vi "CAEN_HVChannel.Create DIM Services.vi"(0 "i ref in":refnum<vi>, 5 "error in":errorcluster) -> (14 "i ref out":refnum<vi>, 19 "error out":errorcluster)   [LabVIEW 2014, in "CAEN_HVChannel.lvlib"]
doc: "This method is used to define the events the object will listen to. Add your own events here."
uses:
  CAEN_HVChannel.lvlib
  CSlibraries-extern/DimLVEvent/LVDimInterface/LVDimInterface.lvlib
  CS_Core/CSSystem/CSSystemLib/CSSystemLib.lvlib
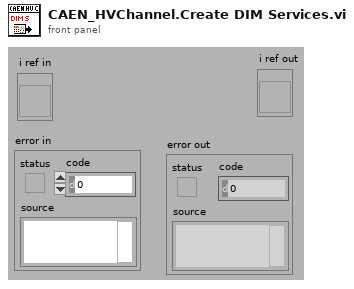
[diagram p1: front panel]
types:
  T1 = typedef "CAEN_HVChannel.lvlib/CAEN_HVChannel.i attribute.ctl" = cluster{"Channel Array":cluster{"Logical Name":string, "Address":string, "error in (no error)":errorcluster, "Name":cluster{"Name":string, "DIM Status":cluster{"no link":bool, "quality":i32, "Time Stamp":timestamp}}, "Status":cluster{"Status":i16, "DIM Status":cluster{"no link":bool, "quality":i32, "Time Stamp":timestamp}}, "V0Set":cluster{"V0Set#EU":cluster{"V0Set#EU":string, "DIM Status":cluster{"no link":bool, "quality":i32, "Time Stamp":timestamp}}, "V0Set":cluster{"V0Set":dbl, "DIM Status":cluster{"no link":bool, "quality":i32, "Time Stamp":timestamp}}, "V0Set#HighEU":cluster{"V0Set#HighEU":dbl, "DIM Status":cluster{"no link":bool, "quality":i32, "Time Stamp":timestamp}}, "V0Set#LowEU":cluster{"V0Set#LowEU":dbl, "DIM Status":cluster{"no link":bool, "quality":i32, "Time Stamp":timestamp}}, "V0Set#Multiplier":dbl}, "I0Set":cluster{"I0Set#EU":cluster{"I0Set#EU":string, "DIM Status":cluster{"no link":bool, "quality":i32, "Time Stamp":timestamp}}, "I0Set":cluster{"I0Set":dbl, "DIM Status":cluster{"no link":bool, "quality":i32, "Time Stamp":timestamp}}, "I0Set#HighEU":cluster{"I0Set#HighEU":dbl, "DIM Status":cluster{"no link":bool, "quality":i32, "Time Stamp":timestamp}}, "I0Set#LowEU":cluster{"I0Set#LowEU":dbl, "DIM Status":cluster{"no link":bool, "quality":i32, "Time Stamp":timestamp}}, "I0Set#Multiplier":dbl}, "V1Set":cluster{"V1Set#EU":cluster{"V1Set#EU":string, "DIM Status":cluster{"no link":bool, "quality":i32, "Time Stamp":timestamp}}, "V1Set":cluster{"V1Set":dbl, "DIM Status":cluster{"no link":bool, "quality":i32, "Time Stamp":timestamp}}, "V1Set#HighEU":cluster{"V1Set#HighEU":dbl, "DIM Status":cluster{"no link":bool, "quality":i32, "Time Stamp":timestamp}}, "V1Set#LowEU":cluster{"V1Set#LowEU":dbl, "DIM Status":cluster{"no link":bool, "quality":i32, "Time Stamp":timestamp}}, "V1Set#Multiplier":dbl}, "I1Set":cluster{"I1Set#EU":cluster{"I1Set#EU":string, "DIM Status":cluster{"no link":bool, "quality":i32, "Time Stamp":timestamp}}, "I1Set":cluster{"I1Set":dbl, "DIM Status":cluster{"no link":bool, "quality":i32, "Time Stamp":timestamp}}, "I1Set#HighEU":cluster{"I1Set#HighEU":dbl, "DIM Status":cluster{"no link":bool, "quality":i32, "Time Stamp":timestamp}}, "I1Set#LowEU":cluster{"I1Set#LowEU":dbl, "DIM Status":cluster{"no link":bool, "quality":i32, "Time Stamp":timestamp}}, "I1Set#Multiplier":dbl}, "RUp":cluster{"RUp#EU":cluster{"RUp#EU":string, "DIM Status":cluster{"no link":bool, "quality":i32, "Time Stamp":timestamp}}, "RUp":cluster{"RUp":dbl, "DIM Status":cluster{"no link":bool, "quality":i32, "Time Stamp":timestamp}}, "RUp#HighEU":cluster{"RUp#HighEU":dbl, "DIM Status":cluster{"no link":bool, "quality":i32, "Time Stamp":timestamp}}, "RUp#LowEU":cluster{"RUp#LowEU":dbl, "DIM Status":cluster{"no link":bool, "quality":i32, "Time Stamp":timestamp}}, "RUp#Multiplier":dbl}, "RDWn":cluster{"RDWn#EU":cluster{"RDWn#EU":string, "DIM Status":cluster{"no link":bool, "quality":i32, "Time Stamp":timestamp}}, "RDWn":cluster{"RDWn":dbl, "DIM Status":cluster{"no link":bool, "quality":i32, "Time Stamp":timestamp}}, "RDWn#HighEU":cluster{"RDWn#HighEU":dbl, "DIM Status":cluster{"no link":bool, "quality":i32, "Time Stamp":timestamp}}, "RDWn#LowEU":cluster{"RDWn#LowEU":dbl, "DIM Status":cluster{"no link":bool, "quality":i32, "Time Stamp":timestamp}}, "RDWn#Multiplier":dbl}, "Trip":cluster{"Trip#EU":cluster{"Trip#EU":string, "DIM Status":cluster{"no link":bool, "quality":i32, "Time Stamp":timestamp}}, "Trip":cluster{"Trip":dbl, "DIM Status":cluster{"no link":bool, "quality":i32, "Time Stamp":timestamp}}, "Trip#HighEU":cluster{"Trip#HighEU":dbl, "DIM Status":cluster{"no link":bool, "quality":i32, "Time Stamp":timestamp}}, "Trip#LowEU":cluster{"Trip#LowEU":dbl, "DIM Status":cluster{"no link":bool, "quality":i32, "Time Stamp":timestamp}}, "Trip#Multiplier":dbl}, "SVMax":cluster{"SVMax#EU":cluster{"SVMax#EU":string, "DIM Status":cluster{"no link":bool, "quality":i32, "Time Stamp":timestamp}}, "SVMax":cluster{"SVMax":dbl, "DIM Status":cluster{"no link":bool, "quality":i32, "Time Stamp":timestamp}}, "SVMax#HighEU":cluster{"SVMax#HighEU":dbl, "DIM Status":cluster{"no link":bool, "quality":i32, "Time Stamp":timestamp}}, "SVMax#LowEU":cluster{"SVMax#LowEU":dbl, "DIM Status":cluster{"no link":bool, "quality":i32, "Time Stamp":timestamp}}, "SVMax#Multiplier":dbl}, "VMon":cluster{"VMon#EU":cluster{"VMon#EU":string, "DIM Status":cluster{"no link":bool, "quality":i32, "Time Stamp":timestamp}}, "VMon":cluster{"VMon":dbl, "DIM Status":cluster{"no link":bool, "quality":i32, "Time Stamp":timestamp}}, "VMon#HighEU":cluster{"VMon#HighEU":dbl, "DIM Status":cluster{"no link":bool, "quality":i32, "Time Stamp":timestamp}}, "VMon#LowEU":cluster{"VMon#LowEU":dbl, "DIM Status":cluster{"no link":bool, "quality":i32, "Time Stamp":timestamp}}, "VMon#Multiplier":dbl}, "IMon":cluster{"IMon#EU":cluster{"IMon#EU":string, "DIM Status":cluster{"no link":bool, "quality":i32, "Time Stamp":timestamp}}, "IMon":cluster{"IMon":dbl, "DIM Status":cluster{"no link":bool, "quality":i32, "Time Stamp":timestamp}}, "IMon#HighEU":cluster{"IMon#HighEU":dbl, "DIM Status":cluster{"no link":bool, "quality":i32, "Time Stamp":timestamp}}, "IMon#LowEU":cluster{"IMon#LowEU":dbl, "DIM Status":cluster{"no link":bool, "quality":i32, "Time Stamp":timestamp}}, "IMon#Multiplier":dbl}, "TripInt":cluster{"TripInt#EU":cluster{"TripInt#EU":string, "DIM Status":cluster{"no link":bool, "quality":i32, "Time Stamp":timestamp}}, "TripInt":cluster{"TripInt":dbl, "DIM Status":cluster{"no link":bool, "quality":i32, "Time Stamp":timestamp}}, "TripInt#HighEU":cluster{"TripInt#HighEU":dbl, "DIM Status":cluster{"no link":bool, "quality":i32, "Time Stamp":timestamp}}, "TripInt#LowEU":cluster{"TripInt#LowEU":dbl, "DIM Status":cluster{"no link":bool, "quality":i32, "Time Stamp":timestamp}}, "TripInt#Multiplier":dbl}, "TripExt":cluster{"TripExt#EU":cluster{"TripExt#EU":string, "DIM Status":cluster{"no link":bool, "quality":i32, "Time Stamp":timestamp}}, "TripExt":cluster{"TripExt":dbl, "DIM Status":cluster{"no link":bool, "quality":i32, "Time Stamp":timestamp}}, "TripExt#HighEU":cluster{"TripExt#HighEU":dbl, "DIM Status":cluster{"no link":bool, "quality":i32, "Time Stamp":timestamp}}, "TripExt#LowEU":cluster{"TripExt#LowEU":dbl, "DIM Status":cluster{"no link":bool, "quality":i32, "Time Stamp":timestamp}}, "TripExt#Multiplier":dbl}, "Pw":cluster{"Pw":cluster{"Pw":bool, "DIM Status":cluster{"no link":bool, "quality":i32, "Time Stamp":timestamp}}, "Pw#CoClose":cluster{"Pw#CoClose":string, "DIM Status":cluster{"no link":bool, "quality":i32, "Time Stamp":timestamp}}, "Pw#CoOpen":cluster{"Pw#CoOpen":string, "DIM Status":cluster{"no link":bool, "quality":i32, "Time Stamp":timestamp}}}, "POn":cluster{"POn":cluster{"POn":bool, "DIM Status":cluster{"no link":bool, "quality":i32, "Time Stamp":timestamp}}, "POn#CoClose":cluster{"POn#CoClose":string, "DIM Status":cluster{"no link":bool, "quality":i32, "Time Stamp":timestamp}}, "POn#CoOpen":cluster{"POn#CoOpen":string, "DIM Status":cluster{"no link":bool, "quality":i32, "Time Stamp":timestamp}}}, "PDwn":cluster{"PDwn":cluster{"PDwn":bool, "DIM Status":cluster{"no link":bool, "quality":i32, "Time Stamp":timestamp}}, "PDwn#CoClose":cluster{"PDwn#CoClose":string, "DIM Status":cluster{"no link":bool, "quality":i32, "Time Stamp":timestamp}}, "PDwn#CoOpen":cluster{"PDwn#CoOpen":string, "DIM Status":cluster{"no link":bool, "quality":i32, "Time Stamp":timestamp}}}, "DIM Service IDs":cluster{"nomV1Set":i32, "nomI1Set":i32, "nomTrip":i32, "nomSVMax":i32, "nomPOn":i32, "nomPDwn":i32, "nomTripInt":i32, "nomTripExt":i32}}[], "VoltageInRangeBand":dbl}
  T2 = cluster{"Logical Name":string, "Address":string, "error in (no error)":errorcluster, "Name":cluster{"Name":string, "DIM Status":cluster{"no link":bool, "quality":i32, "Time Stamp":timestamp}}, "Status":cluster{"Status":i16, "DIM Status":cluster{"no link":bool, "quality":i32, "Time Stamp":timestamp}}, "V0Set":cluster{"V0Set#EU":cluster{"V0Set#EU":string, "DIM Status":cluster{"no link":bool, "quality":i32, "Time Stamp":timestamp}}, "V0Set":cluster{"V0Set":dbl, "DIM Status":cluster{"no link":bool, "quality":i32, "Time Stamp":timestamp}}, "V0Set#HighEU":cluster{"V0Set#HighEU":dbl, "DIM Status":cluster{"no link":bool, "quality":i32, "Time Stamp":timestamp}}, "V0Set#LowEU":cluster{"V0Set#LowEU":dbl, "DIM Status":cluster{"no link":bool, "quality":i32, "Time Stamp":timestamp}}, "V0Set#Multiplier":dbl}, "I0Set":cluster{"I0Set#EU":cluster{"I0Set#EU":string, "DIM Status":cluster{"no link":bool, "quality":i32, "Time Stamp":timestamp}}, "I0Set":cluster{"I0Set":dbl, "DIM Status":cluster{"no link":bool, "quality":i32, "Time Stamp":timestamp}}, "I0Set#HighEU":cluster{"I0Set#HighEU":dbl, "DIM Status":cluster{"no link":bool, "quality":i32, "Time Stamp":timestamp}}, "I0Set#LowEU":cluster{"I0Set#LowEU":dbl, "DIM Status":cluster{"no link":bool, "quality":i32, "Time Stamp":timestamp}}, "I0Set#Multiplier":dbl}, "V1Set":cluster{"V1Set#EU":cluster{"V1Set#EU":string, "DIM Status":cluster{"no link":bool, "quality":i32, "Time Stamp":timestamp}}, "V1Set":cluster{"V1Set":dbl, "DIM Status":cluster{"no link":bool, "quality":i32, "Time Stamp":timestamp}}, "V1Set#HighEU":cluster{"V1Set#HighEU":dbl, "DIM Status":cluster{"no link":bool, "quality":i32, "Time Stamp":timestamp}}, "V1Set#LowEU":cluster{"V1Set#LowEU":dbl, "DIM Status":cluster{"no link":bool, "quality":i32, "Time Stamp":timestamp}}, "V1Set#Multiplier":dbl}, "I1Set":cluster{"I1Set#EU":cluster{"I1Set#EU":string, "DIM Status":cluster{"no link":bool, "quality":i32, "Time Stamp":timestamp}}, "I1Set":cluster{"I1Set":dbl, "DIM Status":cluster{"no link":bool, "quality":i32, "Time Stamp":timestamp}}, "I1Set#HighEU":cluster{"I1Set#HighEU":dbl, "DIM Status":cluster{"no link":bool, "quality":i32, "Time Stamp":timestamp}}, "I1Set#LowEU":cluster{"I1Set#LowEU":dbl, "DIM Status":cluster{"no link":bool, "quality":i32, "Time Stamp":timestamp}}, "I1Set#Multiplier":dbl}, "RUp":cluster{"RUp#EU":cluster{"RUp#EU":string, "DIM Status":cluster{"no link":bool, "quality":i32, "Time Stamp":timestamp}}, "RUp":cluster{"RUp":dbl, "DIM Status":cluster{"no link":bool, "quality":i32, "Time Stamp":timestamp}}, "RUp#HighEU":cluster{"RUp#HighEU":dbl, "DIM Status":cluster{"no link":bool, "quality":i32, "Time Stamp":timestamp}}, "RUp#LowEU":cluster{"RUp#LowEU":dbl, "DIM Status":cluster{"no link":bool, "quality":i32, "Time Stamp":timestamp}}, "RUp#Multiplier":dbl}, "RDWn":cluster{"RDWn#EU":cluster{"RDWn#EU":string, "DIM Status":cluster{"no link":bool, "quality":i32, "Time Stamp":timestamp}}, "RDWn":cluster{"RDWn":dbl, "DIM Status":cluster{"no link":bool, "quality":i32, "Time Stamp":timestamp}}, "RDWn#HighEU":cluster{"RDWn#HighEU":dbl, "DIM Status":cluster{"no link":bool, "quality":i32, "Time Stamp":timestamp}}, "RDWn#LowEU":cluster{"RDWn#LowEU":dbl, "DIM Status":cluster{"no link":bool, "quality":i32, "Time Stamp":timestamp}}, "RDWn#Multiplier":dbl}, "Trip":cluster{"Trip#EU":cluster{"Trip#EU":string, "DIM Status":cluster{"no link":bool, "quality":i32, "Time Stamp":timestamp}}, "Trip":cluster{"Trip":dbl, "DIM Status":cluster{"no link":bool, "quality":i32, "Time Stamp":timestamp}}, "Trip#HighEU":cluster{"Trip#HighEU":dbl, "DIM Status":cluster{"no link":bool, "quality":i32, "Time Stamp":timestamp}}, "Trip#LowEU":cluster{"Trip#LowEU":dbl, "DIM Status":cluster{"no link":bool, "quality":i32, "Time Stamp":timestamp}}, "Trip#Multiplier":dbl}, "SVMax":cluster{"SVMax#EU":cluster{"SVMax#EU":string, "DIM Status":cluster{"no link":bool, "quality":i32, "Time Stamp":timestamp}}, "SVMax":cluster{"SVMax":dbl, "DIM Status":cluster{"no link":bool, "quality":i32, "Time Stamp":timestamp}}, "SVMax#HighEU":cluster{"SVMax#HighEU":dbl, "DIM Status":cluster{"no link":bool, "quality":i32, "Time Stamp":timestamp}}, "SVMax#LowEU":cluster{"SVMax#LowEU":dbl, "DIM Status":cluster{"no link":bool, "quality":i32, "Time Stamp":timestamp}}, "SVMax#Multiplier":dbl}, "VMon":cluster{"VMon#EU":cluster{"VMon#EU":string, "DIM Status":cluster{"no link":bool, "quality":i32, "Time Stamp":timestamp}}, "VMon":cluster{"VMon":dbl, "DIM Status":cluster{"no link":bool, "quality":i32, "Time Stamp":timestamp}}, "VMon#HighEU":cluster{"VMon#HighEU":dbl, "DIM Status":cluster{"no link":bool, "quality":i32, "Time Stamp":timestamp}}, "VMon#LowEU":cluster{"VMon#LowEU":dbl, "DIM Status":cluster{"no link":bool, "quality":i32, "Time Stamp":timestamp}}, "VMon#Multiplier":dbl}, "IMon":cluster{"IMon#EU":cluster{"IMon#EU":string, "DIM Status":cluster{"no link":bool, "quality":i32, "Time Stamp":timestamp}}, "IMon":cluster{"IMon":dbl, "DIM Status":cluster{"no link":bool, "quality":i32, "Time Stamp":timestamp}}, "IMon#HighEU":cluster{"IMon#HighEU":dbl, "DIM Status":cluster{"no link":bool, "quality":i32, "Time Stamp":timestamp}}, "IMon#LowEU":cluster{"IMon#LowEU":dbl, "DIM Status":cluster{"no link":bool, "quality":i32, "Time Stamp":timestamp}}, "IMon#Multiplier":dbl}, "TripInt":cluster{"TripInt#EU":cluster{"TripInt#EU":string, "DIM Status":cluster{"no link":bool, "quality":i32, "Time Stamp":timestamp}}, "TripInt":cluster{"TripInt":dbl, "DIM Status":cluster{"no link":bool, "quality":i32, "Time Stamp":timestamp}}, "TripInt#HighEU":cluster{"TripInt#HighEU":dbl, "DIM Status":cluster{"no link":bool, "quality":i32, "Time Stamp":timestamp}}, "TripInt#LowEU":cluster{"TripInt#LowEU":dbl, "DIM Status":cluster{"no link":bool, "quality":i32, "Time Stamp":timestamp}}, "TripInt#Multiplier":dbl}, "TripExt":cluster{"TripExt#EU":cluster{"TripExt#EU":string, "DIM Status":cluster{"no link":bool, "quality":i32, "Time Stamp":timestamp}}, "TripExt":cluster{"TripExt":dbl, "DIM Status":cluster{"no link":bool, "quality":i32, "Time Stamp":timestamp}}, "TripExt#HighEU":cluster{"TripExt#HighEU":dbl, "DIM Status":cluster{"no link":bool, "quality":i32, "Time Stamp":timestamp}}, "TripExt#LowEU":cluster{"TripExt#LowEU":dbl, "DIM Status":cluster{"no link":bool, "quality":i32, "Time Stamp":timestamp}}, "TripExt#Multiplier":dbl}, "Pw":cluster{"Pw":cluster{"Pw":bool, "DIM Status":cluster{"no link":bool, "quality":i32, "Time Stamp":timestamp}}, "Pw#CoClose":cluster{"Pw#CoClose":string, "DIM Status":cluster{"no link":bool, "quality":i32, "Time Stamp":timestamp}}, "Pw#CoOpen":cluster{"Pw#CoOpen":string, "DIM Status":cluster{"no link":bool, "quality":i32, "Time Stamp":timestamp}}}, "POn":cluster{"POn":cluster{"POn":bool, "DIM Status":cluster{"no link":bool, "quality":i32, "Time Stamp":timestamp}}, "POn#CoClose":cluster{"POn#CoClose":string, "DIM Status":cluster{"no link":bool, "quality":i32, "Time Stamp":timestamp}}, "POn#CoOpen":cluster{"POn#CoOpen":string, "DIM Status":cluster{"no link":bool, "quality":i32, "Time Stamp":timestamp}}}, "PDwn":cluster{"PDwn":cluster{"PDwn":bool, "DIM Status":cluster{"no link":bool, "quality":i32, "Time Stamp":timestamp}}, "PDwn#CoClose":cluster{"PDwn#CoClose":string, "DIM Status":cluster{"no link":bool, "quality":i32, "Time Stamp":timestamp}}, "PDwn#CoOpen":cluster{"PDwn#CoOpen":string, "DIM Status":cluster{"no link":bool, "quality":i32, "Time Stamp":timestamp}}}, "DIM Service IDs":cluster{"nomV1Set":i32, "nomI1Set":i32, "nomTrip":i32, "nomSVMax":i32, "nomPOn":i32, "nomPDwn":i32, "nomTripInt":i32, "nomTripExt":i32}}[]
  T3 = cluster{"Logical Name":string, "Address":string, "error in (no error)":errorcluster, "Name":cluster{"Name":string, "DIM Status":cluster{"no link":bool, "quality":i32, "Time Stamp":timestamp}}, "Status":cluster{"Status":i16, "DIM Status":cluster{"no link":bool, "quality":i32, "Time Stamp":timestamp}}, "V0Set":cluster{"V0Set#EU":cluster{"V0Set#EU":string, "DIM Status":cluster{"no link":bool, "quality":i32, "Time Stamp":timestamp}}, "V0Set":cluster{"V0Set":dbl, "DIM Status":cluster{"no link":bool, "quality":i32, "Time Stamp":timestamp}}, "V0Set#HighEU":cluster{"V0Set#HighEU":dbl, "DIM Status":cluster{"no link":bool, "quality":i32, "Time Stamp":timestamp}}, "V0Set#LowEU":cluster{"V0Set#LowEU":dbl, "DIM Status":cluster{"no link":bool, "quality":i32, "Time Stamp":timestamp}}, "V0Set#Multiplier":dbl}, "I0Set":cluster{"I0Set#EU":cluster{"I0Set#EU":string, "DIM Status":cluster{"no link":bool, "quality":i32, "Time Stamp":timestamp}}, "I0Set":cluster{"I0Set":dbl, "DIM Status":cluster{"no link":bool, "quality":i32, "Time Stamp":timestamp}}, "I0Set#HighEU":cluster{"I0Set#HighEU":dbl, "DIM Status":cluster{"no link":bool, "quality":i32, "Time Stamp":timestamp}}, "I0Set#LowEU":cluster{"I0Set#LowEU":dbl, "DIM Status":cluster{"no link":bool, "quality":i32, "Time Stamp":timestamp}}, "I0Set#Multiplier":dbl}, "V1Set":cluster{"V1Set#EU":cluster{"V1Set#EU":string, "DIM Status":cluster{"no link":bool, "quality":i32, "Time Stamp":timestamp}}, "V1Set":cluster{"V1Set":dbl, "DIM Status":cluster{"no link":bool, "quality":i32, "Time Stamp":timestamp}}, "V1Set#HighEU":cluster{"V1Set#HighEU":dbl, "DIM Status":cluster{"no link":bool, "quality":i32, "Time Stamp":timestamp}}, "V1Set#LowEU":cluster{"V1Set#LowEU":dbl, "DIM Status":cluster{"no link":bool, "quality":i32, "Time Stamp":timestamp}}, "V1Set#Multiplier":dbl}, "I1Set":cluster{"I1Set#EU":cluster{"I1Set#EU":string, "DIM Status":cluster{"no link":bool, "quality":i32, "Time Stamp":timestamp}}, "I1Set":cluster{"I1Set":dbl, "DIM Status":cluster{"no link":bool, "quality":i32, "Time Stamp":timestamp}}, "I1Set#HighEU":cluster{"I1Set#HighEU":dbl, "DIM Status":cluster{"no link":bool, "quality":i32, "Time Stamp":timestamp}}, "I1Set#LowEU":cluster{"I1Set#LowEU":dbl, "DIM Status":cluster{"no link":bool, "quality":i32, "Time Stamp":timestamp}}, "I1Set#Multiplier":dbl}, "RUp":cluster{"RUp#EU":cluster{"RUp#EU":string, "DIM Status":cluster{"no link":bool, "quality":i32, "Time Stamp":timestamp}}, "RUp":cluster{"RUp":dbl, "DIM Status":cluster{"no link":bool, "quality":i32, "Time Stamp":timestamp}}, "RUp#HighEU":cluster{"RUp#HighEU":dbl, "DIM Status":cluster{"no link":bool, "quality":i32, "Time Stamp":timestamp}}, "RUp#LowEU":cluster{"RUp#LowEU":dbl, "DIM Status":cluster{"no link":bool, "quality":i32, "Time Stamp":timestamp}}, "RUp#Multiplier":dbl}, "RDWn":cluster{"RDWn#EU":cluster{"RDWn#EU":string, "DIM Status":cluster{"no link":bool, "quality":i32, "Time Stamp":timestamp}}, "RDWn":cluster{"RDWn":dbl, "DIM Status":cluster{"no link":bool, "quality":i32, "Time Stamp":timestamp}}, "RDWn#HighEU":cluster{"RDWn#HighEU":dbl, "DIM Status":cluster{"no link":bool, "quality":i32, "Time Stamp":timestamp}}, "RDWn#LowEU":cluster{"RDWn#LowEU":dbl, "DIM Status":cluster{"no link":bool, "quality":i32, "Time Stamp":timestamp}}, "RDWn#Multiplier":dbl}, "Trip":cluster{"Trip#EU":cluster{"Trip#EU":string, "DIM Status":cluster{"no link":bool, "quality":i32, "Time Stamp":timestamp}}, "Trip":cluster{"Trip":dbl, "DIM Status":cluster{"no link":bool, "quality":i32, "Time Stamp":timestamp}}, "Trip#HighEU":cluster{"Trip#HighEU":dbl, "DIM Status":cluster{"no link":bool, "quality":i32, "Time Stamp":timestamp}}, "Trip#LowEU":cluster{"Trip#LowEU":dbl, "DIM Status":cluster{"no link":bool, "quality":i32, "Time Stamp":timestamp}}, "Trip#Multiplier":dbl}, "SVMax":cluster{"SVMax#EU":cluster{"SVMax#EU":string, "DIM Status":cluster{"no link":bool, "quality":i32, "Time Stamp":timestamp}}, "SVMax":cluster{"SVMax":dbl, "DIM Status":cluster{"no link":bool, "quality":i32, "Time Stamp":timestamp}}, "SVMax#HighEU":cluster{"SVMax#HighEU":dbl, "DIM Status":cluster{"no link":bool, "quality":i32, "Time Stamp":timestamp}}, "SVMax#LowEU":cluster{"SVMax#LowEU":dbl, "DIM Status":cluster{"no link":bool, "quality":i32, "Time Stamp":timestamp}}, "SVMax#Multiplier":dbl}, "VMon":cluster{"VMon#EU":cluster{"VMon#EU":string, "DIM Status":cluster{"no link":bool, "quality":i32, "Time Stamp":timestamp}}, "VMon":cluster{"VMon":dbl, "DIM Status":cluster{"no link":bool, "quality":i32, "Time Stamp":timestamp}}, "VMon#HighEU":cluster{"VMon#HighEU":dbl, "DIM Status":cluster{"no link":bool, "quality":i32, "Time Stamp":timestamp}}, "VMon#LowEU":cluster{"VMon#LowEU":dbl, "DIM Status":cluster{"no link":bool, "quality":i32, "Time Stamp":timestamp}}, "VMon#Multiplier":dbl}, "IMon":cluster{"IMon#EU":cluster{"IMon#EU":string, "DIM Status":cluster{"no link":bool, "quality":i32, "Time Stamp":timestamp}}, "IMon":cluster{"IMon":dbl, "DIM Status":cluster{"no link":bool, "quality":i32, "Time Stamp":timestamp}}, "IMon#HighEU":cluster{"IMon#HighEU":dbl, "DIM Status":cluster{"no link":bool, "quality":i32, "Time Stamp":timestamp}}, "IMon#LowEU":cluster{"IMon#LowEU":dbl, "DIM Status":cluster{"no link":bool, "quality":i32, "Time Stamp":timestamp}}, "IMon#Multiplier":dbl}, "TripInt":cluster{"TripInt#EU":cluster{"TripInt#EU":string, "DIM Status":cluster{"no link":bool, "quality":i32, "Time Stamp":timestamp}}, "TripInt":cluster{"TripInt":dbl, "DIM Status":cluster{"no link":bool, "quality":i32, "Time Stamp":timestamp}}, "TripInt#HighEU":cluster{"TripInt#HighEU":dbl, "DIM Status":cluster{"no link":bool, "quality":i32, "Time Stamp":timestamp}}, "TripInt#LowEU":cluster{"TripInt#LowEU":dbl, "DIM Status":cluster{"no link":bool, "quality":i32, "Time Stamp":timestamp}}, "TripInt#Multiplier":dbl}, "TripExt":cluster{"TripExt#EU":cluster{"TripExt#EU":string, "DIM Status":cluster{"no link":bool, "quality":i32, "Time Stamp":timestamp}}, "TripExt":cluster{"TripExt":dbl, "DIM Status":cluster{"no link":bool, "quality":i32, "Time Stamp":timestamp}}, "TripExt#HighEU":cluster{"TripExt#HighEU":dbl, "DIM Status":cluster{"no link":bool, "quality":i32, "Time Stamp":timestamp}}, "TripExt#LowEU":cluster{"TripExt#LowEU":dbl, "DIM Status":cluster{"no link":bool, "quality":i32, "Time Stamp":timestamp}}, "TripExt#Multiplier":dbl}, "Pw":cluster{"Pw":cluster{"Pw":bool, "DIM Status":cluster{"no link":bool, "quality":i32, "Time Stamp":timestamp}}, "Pw#CoClose":cluster{"Pw#CoClose":string, "DIM Status":cluster{"no link":bool, "quality":i32, "Time Stamp":timestamp}}, "Pw#CoOpen":cluster{"Pw#CoOpen":string, "DIM Status":cluster{"no link":bool, "quality":i32, "Time Stamp":timestamp}}}, "POn":cluster{"POn":cluster{"POn":bool, "DIM Status":cluster{"no link":bool, "quality":i32, "Time Stamp":timestamp}}, "POn#CoClose":cluster{"POn#CoClose":string, "DIM Status":cluster{"no link":bool, "quality":i32, "Time Stamp":timestamp}}, "POn#CoOpen":cluster{"POn#CoOpen":string, "DIM Status":cluster{"no link":bool, "quality":i32, "Time Stamp":timestamp}}}, "PDwn":cluster{"PDwn":cluster{"PDwn":bool, "DIM Status":cluster{"no link":bool, "quality":i32, "Time Stamp":timestamp}}, "PDwn#CoClose":cluster{"PDwn#CoClose":string, "DIM Status":cluster{"no link":bool, "quality":i32, "Time Stamp":timestamp}}, "PDwn#CoOpen":cluster{"PDwn#CoOpen":string, "DIM Status":cluster{"no link":bool, "quality":i32, "Time Stamp":timestamp}}}, "DIM Service IDs":cluster{"nomV1Set":i32, "nomI1Set":i32, "nomTrip":i32, "nomSVMax":i32, "nomPOn":i32, "nomPDwn":i32, "nomTripInt":i32, "nomTripExt":i32}}
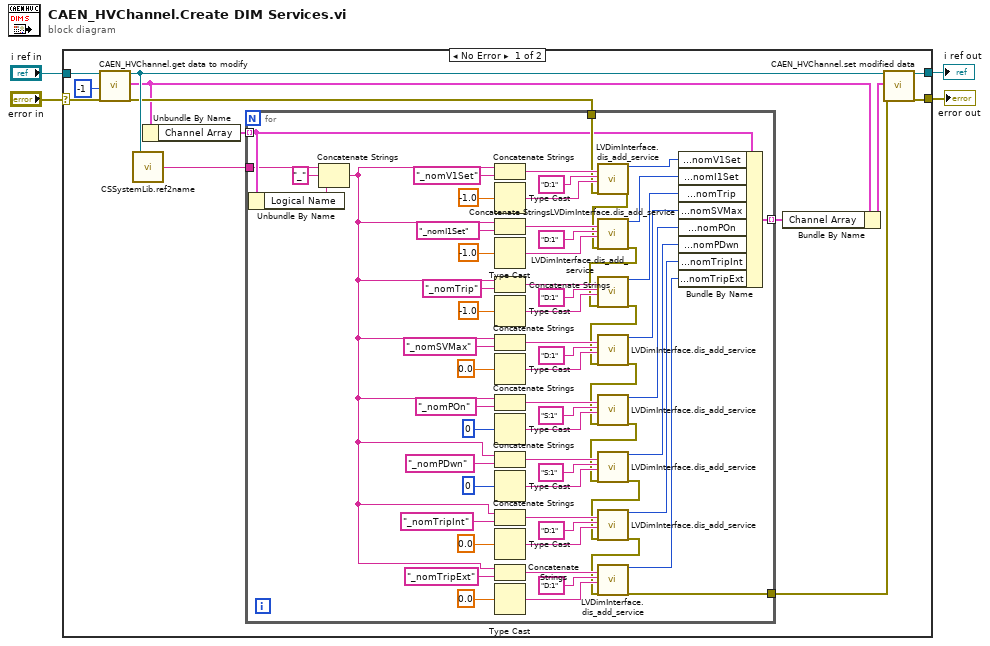
[diagram p0: block diagram]
diagram:
  n1 = case shown="No Error" "error in" {
    selector: "error in" -> [w16 w81]
    tunnel: "i ref in" -> [w17 w82]
    tunnel: [w13 w81] -> w3
    tunnel: [w14 w82] -> w2
    frame No Error {
      n2 = call "CAEN_HVChannel.get data to modify.vi"("i ref in"=w17, "ms timeout (10000)"=-1, "error in (no error)"=w16) -> ("i ref out"=w12:refnum<vi>, "i attribute"=w7:T1, "error out"=w11:errorcluster)  [unwired: 13 in, 1 out]
      n3 = call "CSSystemLib.ref2name.vi"("obj refnum"=w12) -> ("name"=w9:string)
      n4 = Unbundle By Name(w7) -> ("Channel Array"=w6:T2)
      n5 = for {
        tunnel: w11 -> [w75]
        tunnel: [w18] -> w10
        tunnel: w9 -> [w52]
        tunnel: w6 -> [w53] mode=indexing
        tunnel: [w54] -> w5 mode=indexing
        n6 = Unbundle By Name(w53) -> ("Logical Name"=w19:string)
        n7 = Concatenate Strings(w52, "_" ("string"), w19) -> (w23:string)
        n8 = Concatenate Strings(w23, "_nomV1Set" ("string")) -> (w76:string)
        n9 = Type Cast(x=-1.0) -> (*(type *) &x=w80:string)  [unwired: 1 in]
        n10 = Concatenate Strings(w23, "_nomI1Set" ("string")) -> (w73:string)
        n11 = Type Cast(x=-1.0) -> (*(type *) &x=w69:string)  [unwired: 1 in]
        n12 = Concatenate Strings(w23, "_nomTrip" ("string")) -> (w63:string)
        n13 = Type Cast(x=-1.0) -> (*(type *) &x=w67:string)  [unwired: 1 in]
        n14 = Concatenate Strings(w23, "_nomSVMax" ("string")) -> (w48:string)
        n15 = Type Cast(x=0.0) -> (*(type *) &x=w47:string)  [unwired: 1 in]
        n16 = Concatenate Strings(w23, "_nomPOn" ("string")) -> (w58:string)
        n17 = Type Cast(x=i16 0) -> (*(type *) &x=w59:string)  [unwired: 1 in]
        n18 = Concatenate Strings(w23, "_nomPDwn" ("string")) -> (w39:string)
        n19 = Type Cast(x=i16 0) -> (*(type *) &x=w40:string)  [unwired: 1 in]
        n20 = Concatenate Strings(w23, "_nomTripInt" ("string")) -> (w33:string)
        n21 = Type Cast(x=0.0) -> (*(type *) &x=w34:string)  [unwired: 1 in]
        n22 = Concatenate Strings(w23, "_nomTripExt" ("string")) -> (w26:string)
        n23 = Type Cast(x=0.0) -> (*(type *) &x=w27:string)  [unwired: 1 in]
        n24 = call "LVDimInterface.dis_add_service.vi"("serviceName"=w76, "typeDescriptor"="D:1", "data"=w80, "error in (no error)"=w75) -> ("my_serviceID"=w74:i32, "error out"=w68:errorcluster)  [unwired: 14 in]
        n25 = call "LVDimInterface.dis_add_service.vi"("serviceName"=w73, "typeDescriptor"="D:1", "data"=w69, "error in (no error)"=w68) -> ("my_serviceID"=w56:i32, "error out"=w62:errorcluster)  [unwired: 14 in]
        n26 = call "LVDimInterface.dis_add_service.vi"("serviceName"=w63, "typeDescriptor"="D:1", "data"=w67, "error in (no error)"=w62) -> ("my_serviceID"=w55:i32, "error out"=w44:errorcluster)  [unwired: 14 in]
        n27 = call "LVDimInterface.dis_add_service.vi"("serviceName"=w48, "typeDescriptor"="D:1", "data"=w47, "error in (no error)"=w44) -> ("my_serviceID"=w22:i32, "error out"=w43:errorcluster)  [unwired: 14 in]
        n28 = call "LVDimInterface.dis_add_service.vi"("serviceName"=w58, "typeDescriptor"="S:1", "data"=w59, "error in (no error)"=w43) -> ("my_serviceID"=w50:i32, "error out"=w37:errorcluster)  [unwired: 14 in]
        n29 = call "LVDimInterface.dis_add_service.vi"("serviceName"=w39, "typeDescriptor"="S:1", "data"=w40, "error in (no error)"=w37) -> ("my_serviceID"=w21:i32, "error out"=w30:errorcluster)  [unwired: 14 in]
        n30 = call "LVDimInterface.dis_add_service.vi"("serviceName"=w33, "typeDescriptor"="D:1", "data"=w34, "error in (no error)"=w30) -> ("my_serviceID"=w31:i32, "error out"=w24:errorcluster)  [unwired: 14 in]
        n31 = call "LVDimInterface.dis_add_service.vi"("serviceName"=w26, "typeDescriptor"="D:1", "data"=w27, "error in (no error)"=w24) -> ("my_serviceID"=w20:i32, "error out"=w18:errorcluster)  [unwired: 14 in]
        n32 = Bundle By Name(cluster=w53, "DIM Service IDs.nomV1Set"=w74, "DIM Service IDs.nomI1Set"=w56, "DIM Service IDs.nomTrip"=w55, "DIM Service IDs.nomSVMax"=w22, "DIM Service IDs.nomPOn"=w50, "DIM Service IDs.nomPDwn"=w21, "DIM Service IDs.nomTripInt"=w31, "DIM Service IDs.nomTripExt"=w20) -> (w54:T3)
      }
      n33 = Bundle By Name(cluster=w7, "Channel Array"=w5) -> (w8:T1)
      n34 = call "CAEN_HVChannel.set modified data.vi"("i ref in"=w12, "i attribute"=w8, "error in (no error)"=w10) -> ("i ref out"=w14:refnum<vi>, "error out"=w13:errorcluster)  [unwired: 15 in]
    }
    frame Error {
    }
  }
  "i ref out" <- w2
  "error out" <- w3
